vi "File-Locations-Global.vi"() -> ()   [LabVIEW 2014]
panel:
  in  "RAID root path":path
  in  "Directory of last acquisition file accessed":path
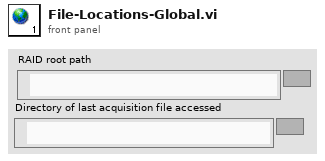
[diagram p1: front panel]
diagram:
